vi "pmu_Check Frame Size.vi"(8 "error in (no error)":errorcluster, 11 "frame size":i32) -> (0 "error out":errorcluster)   [LabVIEW 2013, in "NI_EP_PMU.lvlib"]
uses:
  <vilib>/addons/Electrical Power/PMU/NI_EP_PMU.lvlib
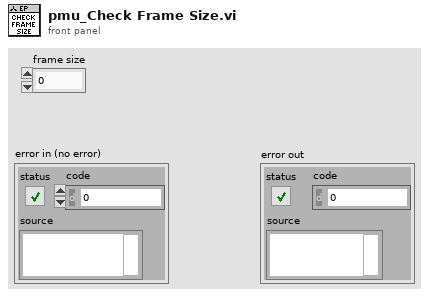
[diagram p1: front panel]
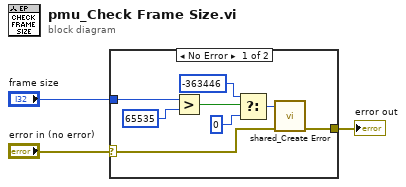
[diagram p0: block diagram]
diagram:
  n1 = case shown="No Error" "error in (no error)" {
    selector: "error in (no error)" -> [w5 w12]
    tunnel: [w6 w12] -> w3
    tunnel: "frame size" -> [w4 _]
    frame No Error {
      n2 = Greater?(x=w4, y=65535) -> (0:w9:bool)
      n3 = Select(t=-363446 ("error code (0)"), s=w9, f=0) -> (s? t:f=w10:i32)
      n4 = call <vilib>:"shared_Create Error.vi"("error in (no error)"=w5, "error code (0)"=w10) -> ("error out"=w6:errorcluster)  [unwired: 9 in]
    }
    frame Error {
    }
  }
  "error out" <- w3
